vi "Get Hi Dew Pt V.vi"(8 "error in (no error)":errorcluster) -> (0 "error out":errorcluster, 3 "function return":sgl)   [LabVIEW 2009, in "VantagePro.lvlib"]
doc: "DllAccess float _stdcall GetHiDewPt_V(void);"
uses:
  VantagePro.lvlib
  <userlib>/VantagePro/VantagePro.dll
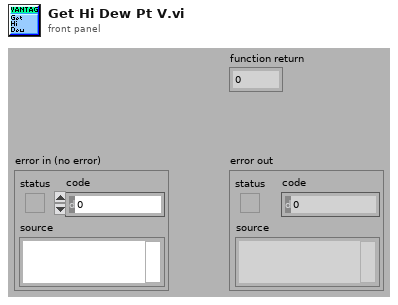
[diagram p1: front panel]
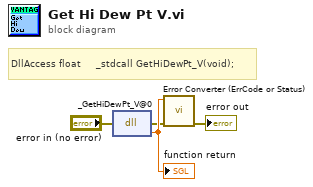
[diagram p0: block diagram]
diagram:
  # "DllAccess float     _stdcall GetHiDewPt_V(void);"
  n1 = dll-call lib="C:/Program Files/National Instruments/LabVIEW 2010/user.lib/VantagePro/VantagePro.*" fn="_GetHiDewPt_V@0"(error in="error in (no error)") -> (error out=w2:errorcluster, w4:sgl)  [unwired: 2 in, 1 out]
  "function return" <- w4
  n2 = call "Error Converter (ErrCode or Status).vi"("error in (no error)"=w2, "error code"=w4) -> ("error out"=→"error out":errorcluster)  [unwired: 9 in]
